vi "bool_to_string.vi"(10 "Boolean":bool) -> (2 "String":string)   [LabVIEW 2016]
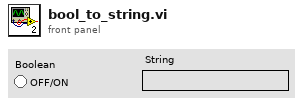
[diagram p1: front panel]
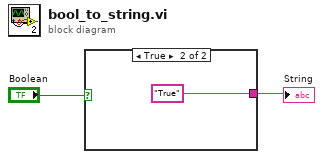
[diagram p0: block diagram]
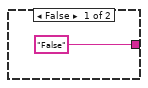
[diagram p2: hidden frame]
diagram:
  n1 = case shown="True" "Boolean" {
    tunnel: ["False" "True"] -> w1
    frame False {
    }
    frame True {
    }
  }
  "String" <- w1
